vi "BNO055 stop receive.vi"(8 "error in (no error)":errorcluster, 11 "y":bool) -> (0 "error out":errorcluster, 3 "Stop_state":bool)   [LabVIEW 2019]
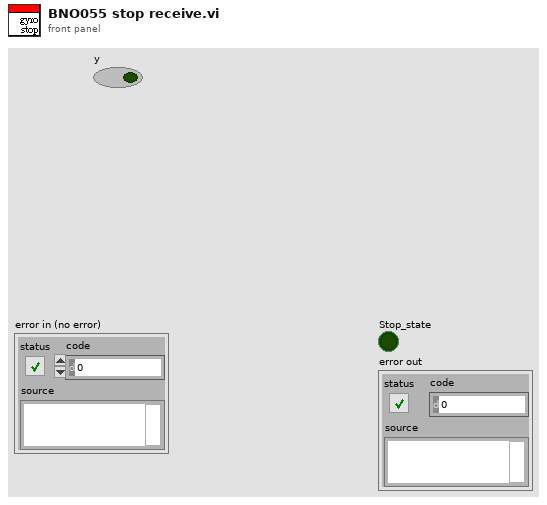
[diagram p1: front panel]
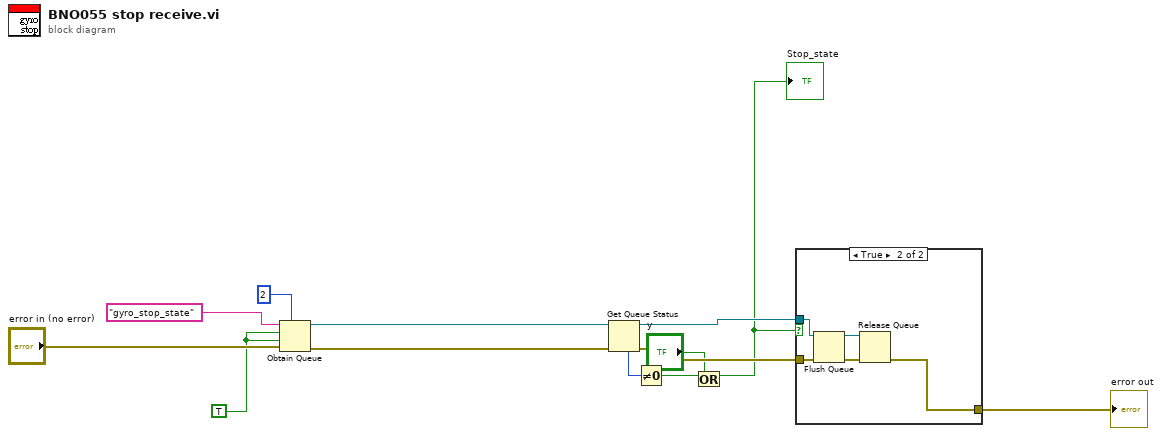
[diagram p0: block diagram]
diagram:
  w3 = TRUE
  n1 = Obtain Queue(max queue size (-1, unlimited)=2, name (unnamed)="gyro_stop_state", element data type=w3, create if not found? (T)=w3, error in (no error)="error in (no error)") -> (queue out=w9:refnum<queue>, error out=w10:errorcluster)  [unwired: 1 out]
  n2 = Get Queue Status(queue=w9, error in (no error)=w10) -> (queue out=w6:refnum<queue>, error out=w5:errorcluster, # elements in queue=w8:i32)  [unwired: 1 in, 5 out]
  n3 = Not Equal To 0?(x=w8) -> (x != 0?=w7:bool)
  n4 = Or(x=w7, y="y") -> (x .or. y?=w2:bool)
  "Stop_state" <- w2
  n5 = case shown="True" w2 {
    tunnel: w6 -> [_ w16]
    tunnel: w5 -> [w14 w19]
    tunnel: [w14 w18] -> w4
    frame False {
    }
    frame True {
      n6 = Flush Queue(queue=w16, error in (no error)=w19) -> (queue out=w15:refnum<queue>, error out=w17:errorcluster)  [unwired: 1 out]
      n7 = Release Queue(queue=w15, error in (no error)=w17) -> (error out=w18:errorcluster)  [unwired: 1 in, 2 out]
    }
  }
  "error out" <- w4
